vi "Read Port Names.vi"(8 "error in (no error)":errorcluster, 11 "Manual Cal Standard in":refnum<class "Cal Standard.lvclass">) -> (0 "error out":errorcluster, 2 "Port Names":string[](array[string]), 3 "Manual Cal Standard out":refnum<class "Cal Standard.lvclass">)   [LabVIEW 2023, in "Manual Cal Standard.lvlib" / "Cal Standard.lvclass"]
uses:
  Cal Standard.lvclass
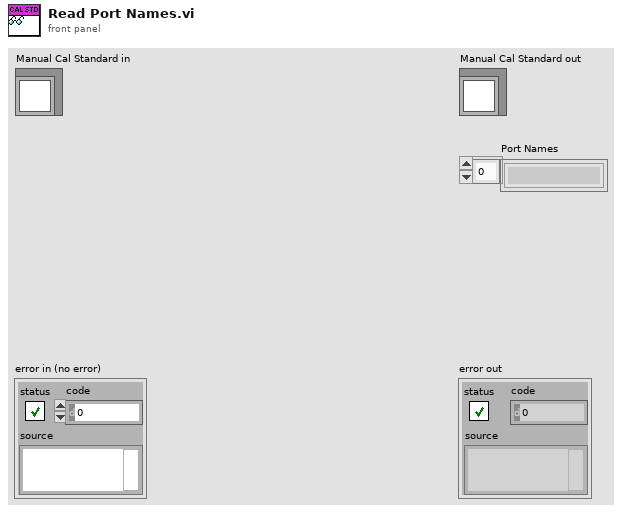
[diagram p1: front panel]
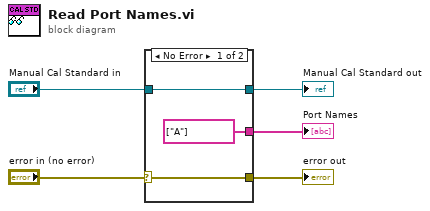
[diagram p0: block diagram]
diagram:
  n1 = case shown="No Error" "error in (no error)" {
    selector: "error in (no error)" -> [w8 w9]
    tunnel: [w8 w9] -> w3
    tunnel: [w7 w10] -> w1
    tunnel: "Manual Cal Standard in" -> [w7 w10]
    tunnel: [string[] ["A"] ("Port Names") _] -> w2
    frame No Error {
    }
    frame Error {
    }
  }
  "error out" <- w3
  "Manual Cal Standard out" <- w1
  "Port Names" <- w2
